vi "komendy.vi"() -> ()   [LabVIEW 2018]
uses:
  <vilib>/NI Modbus.llb/MB Modbus Command.ctl
  <vilib>/NI Modbus.llb/MB Serial Master Query Read Holding Registers (poly).vi
panel:
  out "Registers 2":cluster{"Registers":u16[], "Discrete":bool[]}
  out "Registers":cluster{"Registers":u16[], "Discrete":bool[]}
  in  "Modbus Command":T1={"Function Code"=1, "Starting Address"=0, "Quantity"=0, "Data"=[], "Discrete"=[]} {"Function Code" items=["Read Coils"=1, "Read Discrete Inputs"=2, "Read Holding Registers"=3, "Read Input Registers"=4, "Write Single Coil"=5, "Write Single Register"=6, "Read Exception Status"=7, "Write Multiple Coils"=15, "Write Multiple Registers"=16]}
  out "Holding Registers":u16[](array[numeric])
  in  "Quantity":u16=1
  in  "Starting Address":u16
  in  "Serial Parameters":T2 {"Slave Address" format="%.0x"}
  in  "Mode":enum16{"RTU", "ASCII"}(ring)
  in  "Baud Rate":u32=9600
  out "error out":errorcluster
  in  "error in (no error)":errorcluster
  in  "VISA resource name":refnum<visa-resource-name>
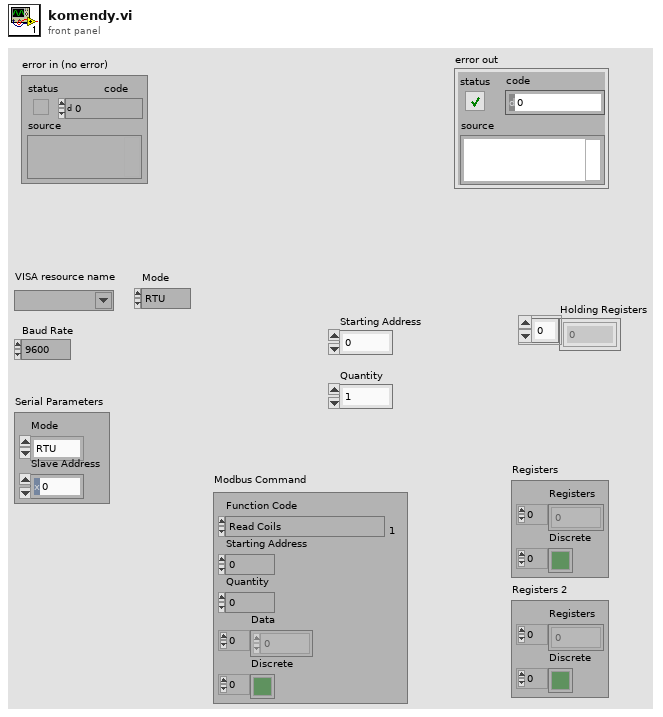
[diagram p1: front panel]
types:
  T1 = typedef "MB Modbus Command.ctl" = cluster{"Function Code":u8, "Starting Address":u16, "Quantity":u16, "Data":u16[], "Discrete":bool[]}
  T2 = cluster{"Mode":enum16{"RTU", "ASCII"}, "Slave Address":u8}
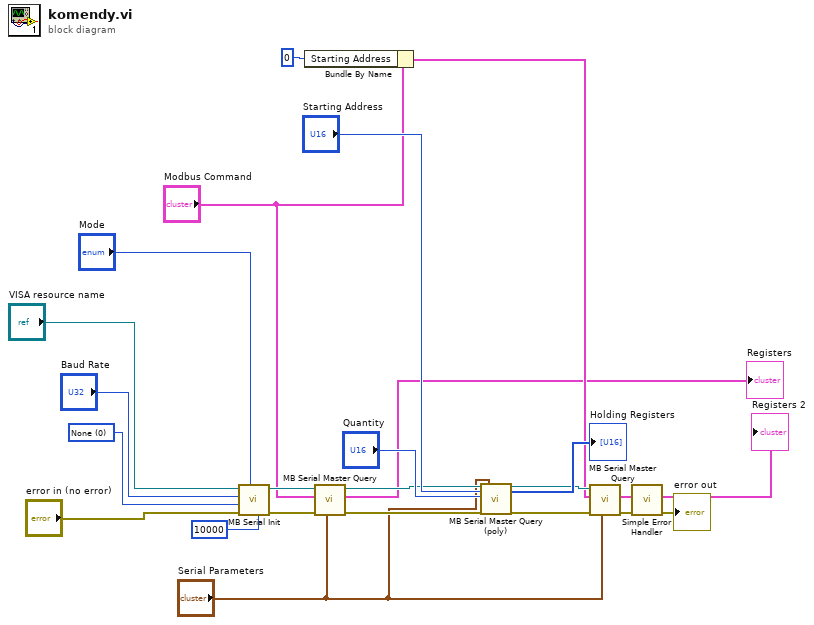
[diagram p0: block diagram]
diagram:
  w18 = u16 0 items=["None", "Odd", "Even", "Mark", "Space"] ("Parity")
  n1 = call <vilib>:"MB Serial Init.vi"("Timeout"=u32 10000, "Mode"="Mode", "error in (no error)"="error in (no error)", "Parity"=w18, "Baud Rate"="Baud Rate", "VISA resource name"="VISA resource name") -> ("error out"=w13:errorcluster, "VISA resource name out"=w12:refnum<visa-resource-name>)  [unwired: 4 in]
  n2 = Bundle By Name(cluster="Modbus Command", "Starting Address"=u16 0) -> (w5:T1)
  n3 = call <vilib>:"MB Serial Master Query.vi"("Serial Parameters"="Serial Parameters", "error in (no error)"=w13, "Modbus Command"="Modbus Command", "VISA resource name"=w12) -> ("error out"=w10:errorcluster, "Registers"=→"Registers":cluster{"Registers":u16[], "Discrete":bool[]}, "VISA resource name out"=w11:refnum<visa-resource-name>)  [unwired: 3 in, 2 out]
  n4 = call-poly <vilib>:"MB Serial Master Query (poly).vi"("VISA resource name"=w11, "Starting Address"="Starting Address", "Quantity"="Quantity", "error in"=w10, "Serial Parameters"="Serial Parameters") -> ("VISA resource name out"=w7:refnum<visa-resource-name>, "Holding Registers"=→"Holding Registers":u16[], "error out"=w8:errorcluster)  [unwired: 11 in, 1 out]
  n5 = call <vilib>:"MB Serial Master Query.vi"("Serial Parameters"="Serial Parameters", "error in (no error)"=w8, "Modbus Command"=w5, "VISA resource name"=w7) -> ("error out"=w9:errorcluster, "Registers"=→"Registers 2":cluster{"Registers":u16[], "Discrete":bool[]})  [unwired: 3 in, 3 out]
  n6 = call <vilib>:"Simple Error Handler.vi"("error in (no error)"=w9) -> ("error out"=→"error out":errorcluster)  [unwired: 4 in, 4 out]
